vi "Ke2000 Reading MilAmp.vi"(8 "error in (no error)":errorcluster, 11 "VISA resource name":refnum<visa-resource-name>) -> (0 "error out":errorcluster, 2 "uA":string, 3 "VISA resource name out":refnum<visa-resource-name>)   [LabVIEW 2009]
panel:
  out "Mili Amp":dbl
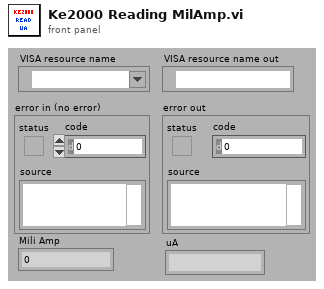
[diagram p1: front panel]
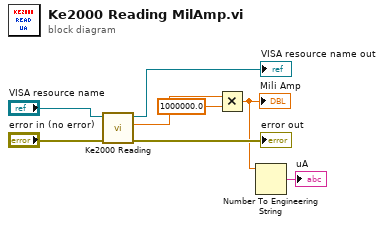
[diagram p0: block diagram]
diagram:
  n1 = call "Ke2000 Reading.vi"("error in (no error)"="error in (no error)", "VISA resource name"="VISA resource name") -> ("error out"=→"error out":errorcluster, "Measurement"=w6:dbl, "VISA resource name out"=→"VISA resource name out":refnum<visa-resource-name>)  [unwired: 6 in, 1 out]
  n2 = Multiply(x=w6, y=1000000.0) -> (x*y=w2:dbl)
  "Mili Amp" <- w2
  n3 = Number To Engineering String(4:w2) -> (0:→"uA":string)  [unwired: 3 in]
